vi "Sample_Scan_Time_Calc.vi"(7 "Speed [micron/s]":dbl=10.0, 8 "Delta M3":dbl, 9 "Delta M1/2 In Plain":dbl, 10 "Line Spacing [microns]":dbl=10.0, 11 "Scan Mode":T1=2 items=["Mode 1", "Mode 2", "Continuous 1", "Continuous 2"]) -> (1 "Scan Time (hous:minutes:seconds)":string, 2 "Scan Time (s)":dbl, 3 "Iterations (N)":i32, 4 "Long Edge Distance (steps)":i32, 6 "Line Spacing (steps)":string="0")   [LabVIEW 2018]
uses:
  Scan Mode.ctl
  ConversionAndInformation/Unit_Control.ctl
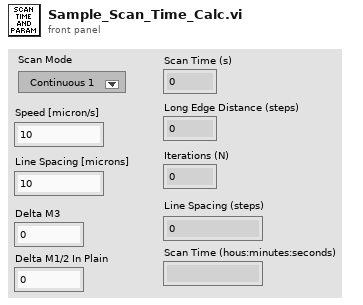
[diagram p1: front panel]
types:
  T1 = typedef "Scan Mode.ctl" = u16
  T2 = typedef "Unit_Control.ctl" = enum16{"Angle (Degrees)", "Rad", "Angle [TMC]", "Microsteps [TMC]", "Inches", "Nanometer", "Meter", "Centimeter", "Millimeter", "Micron"}
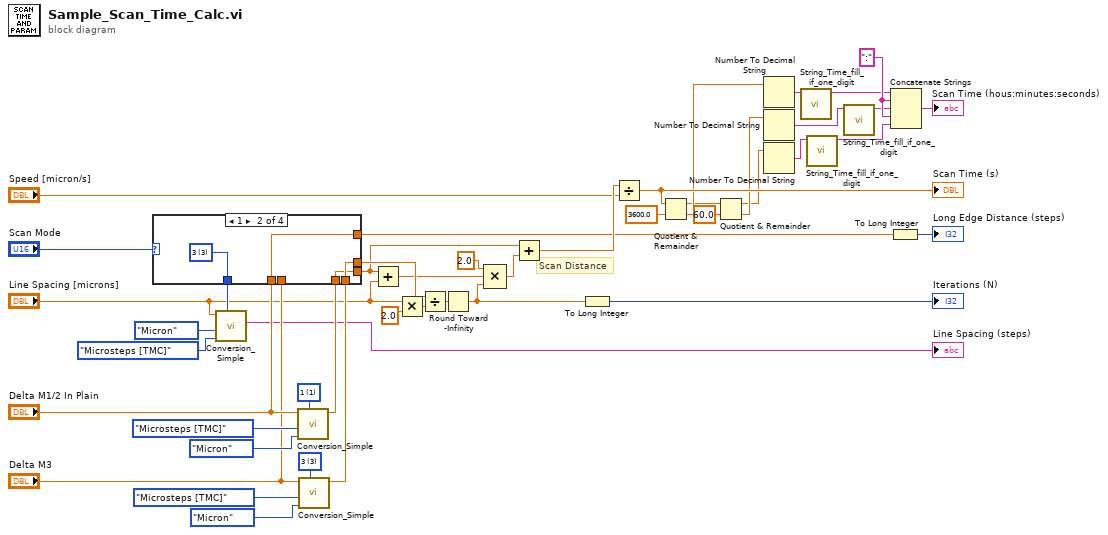
[diagram p0: block diagram]
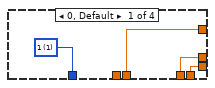
[diagram p2: hidden frame]
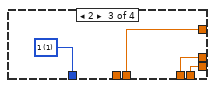
[diagram p3: hidden frame]
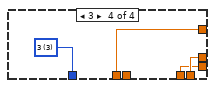
[diagram p4: hidden frame]
diagram:
  w11 = ":"
  w36 = u16 1 items=["none", "1", "2", "3", "4", "all"] ("Motor")
  w37 = u16 3 items=["none", "1", "2", "3", "4", "all"] ("Motor")
  # "Scan Distance"
  n1 = call "Conversion_Simple.vi"("Motor"=w36, "Output Unit"=Unit_Control."Micron", "Input Unit"=Unit_Control."Microsteps [TMC]" ("Output Unit"), "Input"="Delta M1/2 In Plain") -> ("Output"=w35:dbl)  [unwired: 6 in, 1 out]
  n2 = call "Conversion_Simple.vi"("Motor"=w37, "Output Unit"=Unit_Control."Micron", "Input Unit"=Unit_Control."Microsteps [TMC]" ("Output Unit"), "Input"="Delta M3") -> ("Output"=w34:dbl)  [unwired: 6 in, 1 out]
  n3 = case shown="1" "Scan Mode" {
    tunnel: w35 -> [w49 w52 w57 w60]
    tunnel: [w49 w53 w57 w61] -> w45
    tunnel: w34 -> [w48 w53 w56 w61]
    tunnel: [w48 w52 w56 w60] -> w28
    tunnel: "Delta M1/2 In Plain" -> [_ w51 _ w59]
    tunnel: "Delta M3" -> [w47 _ w55 _]
    tunnel: [w47 w51 w55 w59] -> w3
    tunnel: [w46 w50 w54 w58] -> w23
    frame 0, Default {
      w46 = u16 1 items=["none", "1", "2", "3", "4", "all"] ("Motor")
    }
    frame 1 {
      w50 = u16 3 items=["none", "1", "2", "3", "4", "all"] ("Motor")
    }
    frame 2 {
      w54 = u16 1 items=["none", "1", "2", "3", "4", "all"] ("Motor")
    }
    frame 3 {
      w58 = u16 3 items=["none", "1", "2", "3", "4", "all"] ("Motor")
    }
  }
  n4 = call "Conversion_Simple.vi"("Motor"=w23, "Output Unit"=Unit_Control."Microsteps [TMC]", "Input Unit"=Unit_Control."Micron" ("Output Unit"), "Input"="Line Spacing [microns]") -> ("Output"=→"Line Spacing (steps)":string)  [unwired: 6 in, 1 out]
  n5 = Add(x=w28, y="Line Spacing [microns]") -> (x+y=w32:dbl)
  n6 = Multiply(x="Line Spacing [microns]", y=2.0 ("x")) -> (x*y=w42:dbl)
  n7 = Divide(x=w45, y=w42) -> (x/y=w44:dbl)
  n8 = Round Toward -Infinity(1:w44) -> (0:w27:dbl)
  n9 = Compound Arithmetic op=MULTIPLY(2.0 ("value"), w32, w27) -> (w31:dbl)
  n10 = Add(x=w28, y=w31) -> (x+y=w30:dbl)
  n11 = To Long Integer(number=w27) -> (32bit integer=→"Iterations (N)":i32)
  n12 = Divide(x=w30, y="Speed [micron/s]") -> (x/y=w18:dbl)
  "Scan Time (s)" <- w18
  n13 = Quotient & Remainder(x=w18, y=3600.0) -> (x-y*floor(x/y)=w14:dbl, floor(x/y)=w16:dbl)
  n14 = Quotient & Remainder(x=w14, y=60.0) -> (x-y*floor(x/y)=w12:dbl, floor(x/y)=w13:dbl)
  n15 = Number To Decimal String(number=w16) -> (decimal integer string=w9:string)  [unwired: 1 in]
  n16 = Number To Decimal String(number=w13) -> (decimal integer string=w7:string)  [unwired: 1 in]
  n17 = Number To Decimal String(number=w12) -> (decimal integer string=w5:string)  [unwired: 1 in]
  n18 = call "String_Time_fill_if_one_digit.vi"("String"=w9) -> ("String 2"=w8:string)  [unwired: 10 in]
  n19 = call "String_Time_fill_if_one_digit.vi"("String"=w5) -> ("String 2"=w4:string)  [unwired: 10 in]
  n20 = call "String_Time_fill_if_one_digit.vi"("String"=w7) -> ("String 2"=w6:string)  [unwired: 10 in]
  n21 = To Long Integer(number=w3) -> (32bit integer=→"Long Edge Distance (steps)":i32)
  n22 = Concatenate Strings(w8, w11, w6, w11, w4) -> (→"Scan Time (hous:minutes:seconds)":string)
